vi "LSX Set Gripper.vi"(6 "s2":i32, 7 "c2":i32, 8 "error in (no error)":errorcluster, 9 "s1":i32, 10 "c1":i32, 11 "lLSID":i32) -> (0 "error out":errorcluster, 3 "function return":i32)   [LabVIEW 2016, in "Tango_DLL.lvlib"]
doc: "TANGOAPI int TANGOCALL LSX_SetGripper (int lLSID, int c1, int s1, int c2, int s2);"
uses:
  Tango_DLL.lvlib
  2017/Microscope Control/Device Library/Stages/Marzhauser/SCAN IM 120 x 80/Tango DLL VIs/Tango_DLL.dll
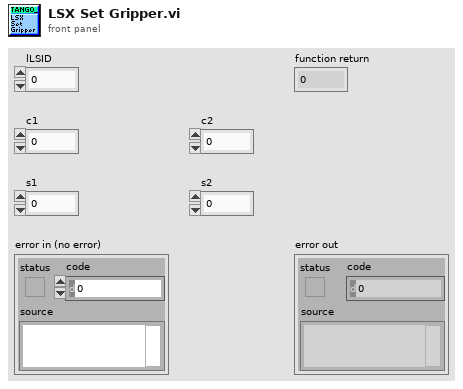
[diagram p1: front panel]
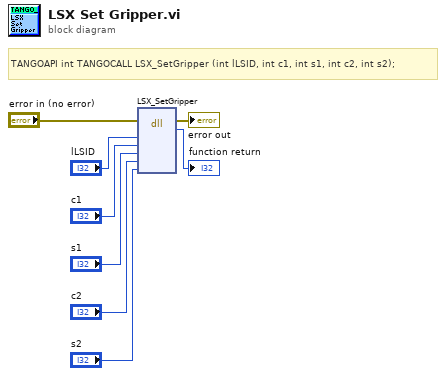
[diagram p0: block diagram]
diagram:
  # "TANGOAPI int TANGOCALL LSX_SetGripper (int lLSID, int c1, int s1, int c2, int s2);"
  n1 = dll-call lib="C:/Users/4PiSMS/Documents/Microscope Control/2017/Microscope Control/Device Library/Stages/Marzhauser/SCAN IM 120 x 80/Tango DLL VIs/Tango_DLL.*" fn="LSX_SetGripper"(error in="error in (no error)", "lLSID"="lLSID", "c1"="c1", "s1"="s1", "c2"="c2", "s2"="s2") -> (error out=→"error out":errorcluster, →"function return":i32)  [unwired: 7 in, 1 out]
